vi "Create Test Configuration.vi"(10 "RIO Device":T1="RIO0") -> (0 "error out":errorcluster, 1 "Names":string[](array[string]), 2 "Line Array":T2[](array[typedef]), 3 "Module Configuration":refnum<class "FPGA Module configuration.lvclass">, 4 "Channels":refnum<class "TBM channel.lvclass">[](array[class]), 5 "instance identifier":string)   [LabVIEW 2014]
doc: "This VI creates a standard test configuration for other unit tests. It currently creates and adds one line with every datatype to the module configuration."
uses:
  <vilib>/NI/Tag Bus Module Framework/channel/channel classification.ctl
  <vilib>/NI/Tag Bus Module Framework/channel/TBM channel.lvclass
  module/configuration/FPGA Module configuration.lvclass
  <vilib>/NI/Configuration Framework/serializable configuration/NISE_CEF_serializable configuration.lvclass
  module/configuration/Line.ctl
  fpga channel/FPGA Channel.lvclass
  <vilib>/NI/Tag Bus/tag/Data Type.ctl
  <vilib>/NI/Tag Bus/tag/tag descriptor.lvclass
  <vilib>/fxp/LVFixedPointRepBitsTypeDef.ctl
  <vilib>/userdefined/High Color/nirio_resource_hc.ctl
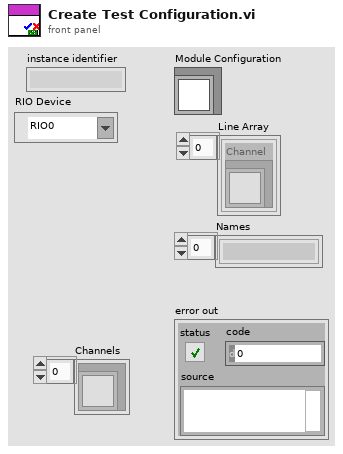
[diagram p1: front panel]
types:
  T1 = typedef "nirio_resource_hc.ctl" = tag
  T2 = typedef "FPGA Module configuration.lvclass/Line.ctl" = cluster{"Channel":refnum<class "FPGA Channel.lvclass">}
  T3 = typedef "LVFixedPointRepBitsTypeDef.ctl" = cluster{"Signed":bool, "Word Length":u32, "Integer Word Length":i32}
  T4 = typedef "tag bus.lvlib/tag descriptor.lvclass/Data Type.ctl" = enum16{"Double", "Single", "I64", "I32", "I16", "I8", "U64", "U32", "U16", "U8", "Boolean", "String", "Array of Double", "Array of Single", "Array of I64", "Array of I32", "Array of I16", "Array of I8", "Array of U64", "Array of U32", "Array of U16", "Array of U8", "Array of Boolean", "Array of String"}
  T5 = typedef "TBM channel.lvclass/channel classification.ctl" = enum16{"input data", "output data", "processing parameter", "processing result"}
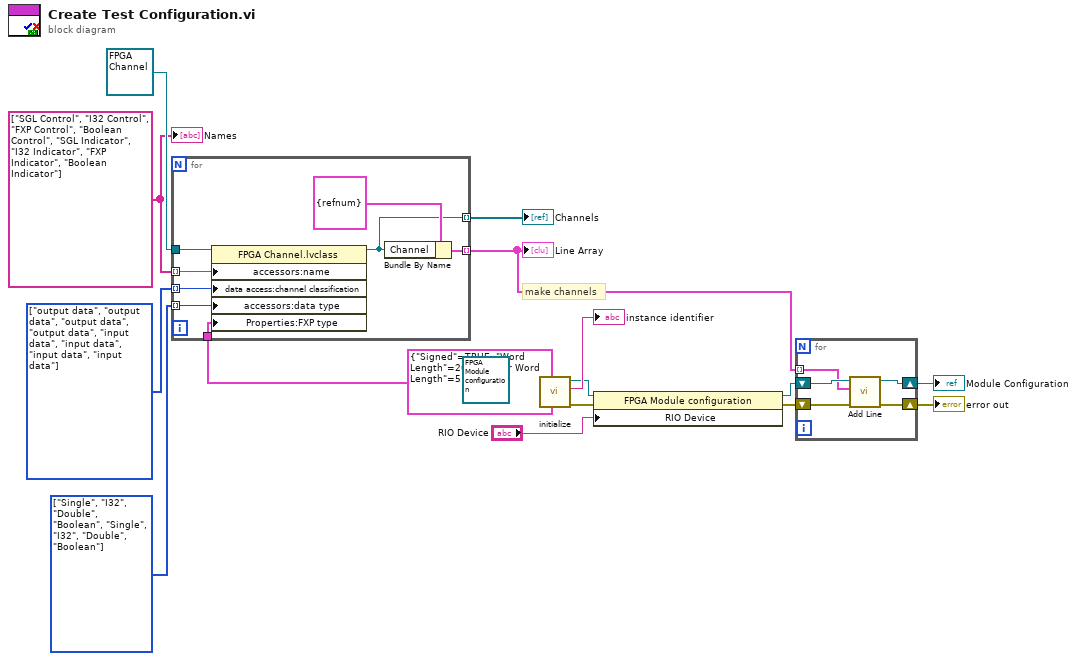
[diagram p0: block diagram]
diagram:
  w2 = T4[] [enum."Single", enum."I32", enum."Double", enum."Boolean", enum."Single", enum."I32", enum."Double", enum."Boolean"] items=["Double", "Single", "I64", "I32", "I16", "I8", "U64", "U32", "U16", "U8", "Boolean", "String", "Array of Double", "Array of Single", "Array of I64", "Array of I32", "Array of I16", "Array of I8", "Array of U64", "Array of U32", "Array of U16", "Array of U8", "Array of Boolean", "Array of String"]
  w3 = T5[] [enum."output data", enum."output data", enum."output data", enum."output data", enum."input data", enum."input data", enum."input data", enum."input data"] items=["input data", "output data", "processing parameter", "processing result"]
  w4 = string[] ["SGL Control", "I32 Control", "FXP Control", "Boolean Control", "SGL Indicator", "I32 Indicator", "FXP Indicator", "Boolean Indicator"]
  # "make channels"
  n1 = for {
    tunnel: w3 -> [w19] mode=indexing
    tunnel: [w21] -> w8 mode=indexing
    tunnel: refnum<class "FPGA Channel.lvclass"> refnum ("Channel") -> [w23]
    tunnel: [w22] -> w5 mode=indexing
    tunnel: w4 -> [w20] mode=indexing
    tunnel: w2 -> [w18] mode=indexing
    tunnel: T3 {"Signed"=TRUE, "Word Length"=20, "Integer Word Length"=5} ("FXP type") -> [w17]
    n2 = property class="FPGA Channel.lvclass"(reference=w23, "accessors:name"=w20, "data access:channel classification"=w19, "accessors:data type"=w18, "Properties:FXP type"=w17) -> (reference out=w21:refnum<class "FPGA Channel.lvclass">)  [unwired: 1 in, 1 out]
    n3 = Bundle By Name(cluster=T2 {"Channel"=refnum} ("Line"), "Channel"=w21) -> (w22:T2)
  }
  "Line Array" <- w5
  "Channels" <- w8
  n4 = call <vilib>:"initialize.vi"("configuration in"=refnum<class "FPGA Module configuration.lvclass"> refnum ("tag bus configurable plugin module configuration")) -> ("error out"=w14:errorcluster, "identifier"=→"instance identifier":string, "configuration out"=w12:refnum<class "FPGA Module configuration.lvclass">)  [unwired: 8 in]
  n5 = property class="FPGA Module configuration"(reference=w12, error in=w14, "RIO Device"="RIO Device") -> (reference out=w9:refnum<class "FPGA Module configuration.lvclass">, error out=w13:errorcluster)
  n6 = for {
    tunnel: w5 -> [w25] mode=indexing
    shift-right: [w28] -> w11
    shift-left: w9 -> [w29]
    shift-right: [w26] -> w16
    shift-left: w13 -> [w27]
    n7 = call "Add Line.vi"("error in"=w27, "Line"=w25, "FPGA Module configuration in"=w29) -> ("error out"=w26:errorcluster, "FPGA Module configuration out"=w28:refnum<class "FPGA Module configuration.lvclass">)  [unwired: 6 in, 1 out]
  }
  "error out" <- w16
  "Module Configuration" <- w11
  "Names" <- w4
